vi "fcs_read.vi"(8 "error in (no error)":errorcluster, 11 "Path":path) -> (0 "error out":errorcluster, 1 "BEGINDATA":i32, 2 "byte offset":i64, 3 "Array":sgl[][](array[numeric]))   [LabVIEW 2013]
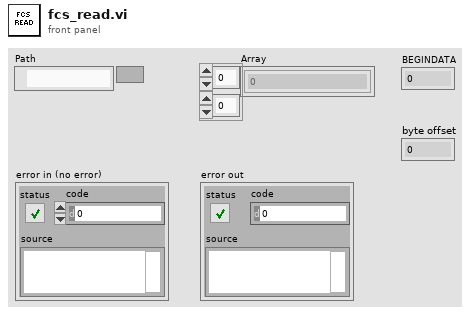
[diagram p1: front panel]
types:
  T1 = enum16{"big-endian, network order", "native, host order", "little-endian"}
  T2 = enum16{"open", "replace", "create", "open or create", "replace or create", "replace or create with confirmation"}
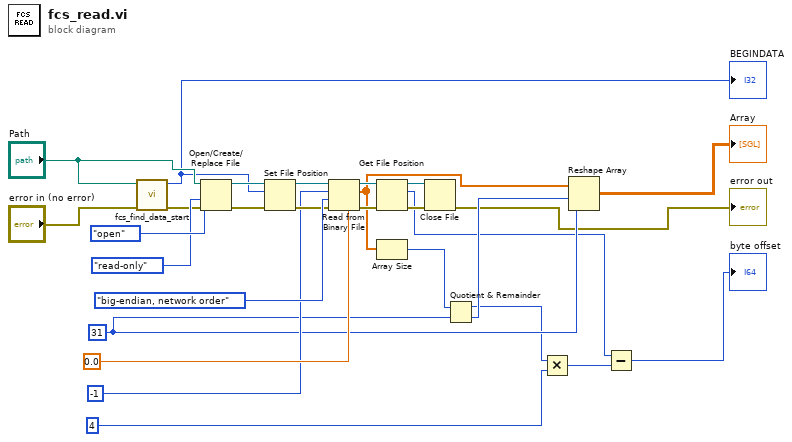
[diagram p0: block diagram]
diagram:
  w9 = 31 ("dimension size")
  n1 = call "fcs_find_data_start.vi"("error in"="error in (no error)", "File Path"="Path") -> ("error out"=w17:errorcluster, "BEGINDATA"=w16:i32)  [unwired: 6 in, 2 out]
  "BEGINDATA" <- w16
  n2 = Open/Create/Replace File(file path (use dialog)="Path", error in=w17, operation (0:open)=T2."open", access (0:read/write)=enum16{"read/write", "read-only", "write-only"}."read-only") -> (refnum out=w21:refnum<file>, error out=w18:errorcluster)  [unwired: 2 in, 1 out]
  n3 = Set File Position(offset (in bytes) (0)=w16, refnum=w21, error in=w18) -> (refnum out=w20:refnum<file>, error out=w19:errorcluster)  [unwired: 1 in]
  n4 = Read from Binary File(5:sgl 0.0, 8:w19, 9:T1."big-endian, network order" ("byte order (0:big-endian, network order)"), 10:-1, 11:w20) -> (0:w15:errorcluster, 2:w10:sgl[], 3:w13:refnum<file>)  [unwired: 1 in, 1 out]
  n5 = Get File Position(4:w15, 7:w13) -> (0:w14:errorcluster, 2:w4:i64, 3:w12:refnum<file>)
  n6 = Array Size(array=w10) -> (size(s)=w8:i32)
  n7 = Close File(refnum=w12, error in=w14) -> (error out=→"error out":errorcluster)  [unwired: 1 out]
  n8 = Quotient & Remainder(x=w8, y=w9) -> (x-y*floor(x/y)=w1:i32, floor(x/y)=w7:i32)
  n9 = Multiply(x=w1, y=4) -> (x*y=w5:i32)
  n10 = Reshape Array(w10, w7, w9) -> (→"Array":sgl[][])
  n11 = Subtract(x=w4, y=w5) -> (x-y=→"byte offset":i64)
